vi "Get Value by Key.vi"(8 "error in (no error)":errorcluster caption="错误输入（无错误）", 10 "Key":string, 11 "Dictionary In":refnum<class "Dictionary.lvclass"> caption="DNL_LabVIEW Object in") -> (0 "error out":errorcluster caption="错误输出", 1 "Key Exist?":bool, 2 "Value":string, 3 "Dictionary Out":refnum<class "Dictionary.lvclass"> caption="DNL_LabVIEW Object out")   [LabVIEW 2012, in "Dictionary.lvclass"]
uses:
  Dictionary.lvclass
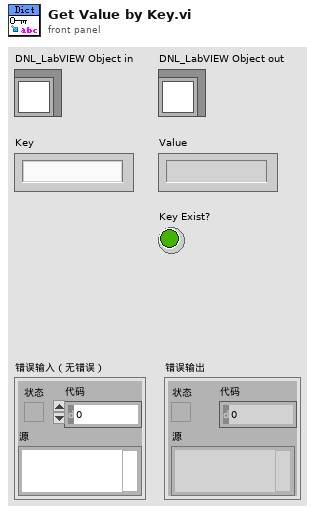
[diagram p1: front panel]
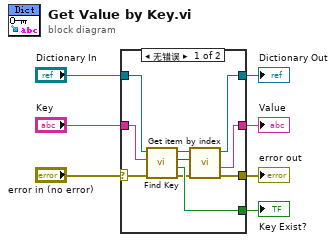
[diagram p0: block diagram]
diagram:
  n1 = case shown="无错误" "error in (no error)" {
    selector: "error in (no error)" -> [w15 w19]
    tunnel: [w10 w19] -> w6
    tunnel: [w11 w18] -> w4
    tunnel: "Dictionary In" -> [w17 w18]
    tunnel: "Key" -> [w16 _]
    tunnel: [w14 _] -> w2
    tunnel: [w9 _] -> w1
    frame No Error {
      n2 = call "Find Key.vi"("error in (no error)"=w15, "Key"=w16, "Dictionary In"=w17) -> ("error out"=w8:errorcluster, "Key Exist?"=w14:bool, "Index"=w12:i32, "Dictionary Out"=w13:refnum<class "Dictionary.lvclass">)  [unwired: 5 in]
      n3 = call "Get item by index.vi"("error in (no error)"=w8, "Index"=w12, "Dictionary In"=w13) -> ("error out"=w10:errorcluster, "Value"=w9:string, "Dictionary Out"=w11:refnum<class "Dictionary.lvclass">)  [unwired: 5 in, 1 out]
    }
    frame Error {
    }
  }
  "error out" <- w6
  "Dictionary Out" <- w4
  "Key Exist?" <- w2
  "Value" <- w1
